vi "AvaSpec Control.vi"(6 "Path":path, 8 "error in (no error)":errorcluster, 9 "Sphere Indicator":T1, 10 "dup Message Queue":refnum<queue>, 11 "VI ref":refnum<vi>) -> (0 "error out":errorcluster)   [LabVIEW 2013]
uses:
  support/Message Queue/Message Cluster.ctl
  Acquisition/Sphere Indicator.ctl
  support/Message Queue/AvaSpec Message Queue.lvlib
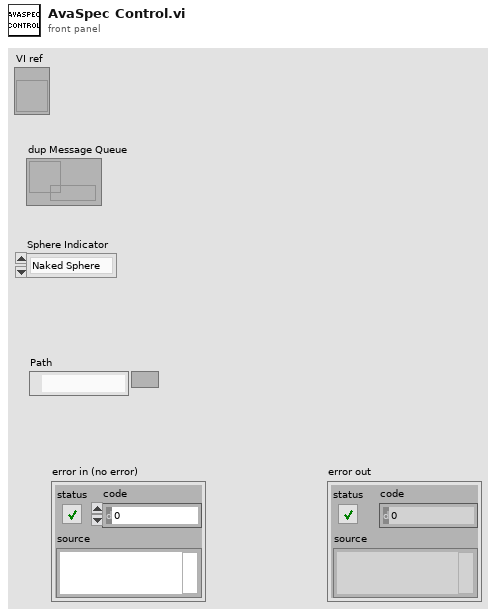
[diagram p1: front panel]
types:
  T1 = typedef "Sphere Indicator.ctl" = enum16{"Naked Sphere", "Insulated Sphere"}
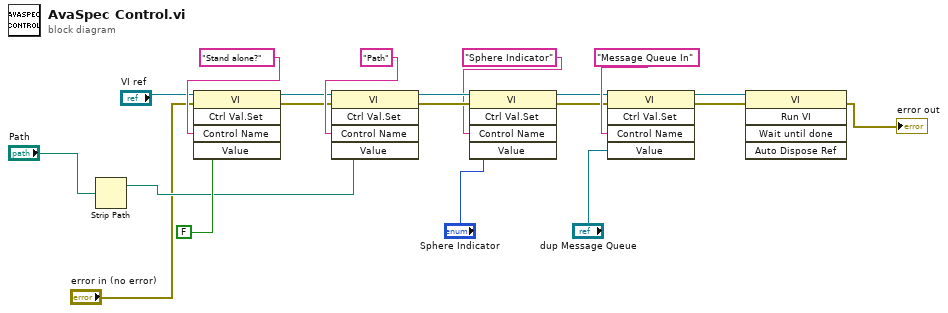
[diagram p0: block diagram]
diagram:
  n1 = Strip Path(path="Path") -> (stripped path=w4:path)  [unwired: 1 out]
  n2 = invoke class="VI" method="Ctrl Val.Set"(reference="VI ref", error in="error in (no error)", "Control Name"="Stand alone?", "Value"=FALSE) -> (reference out=w16:refnum<vi>, error out=w17:errorcluster)  [unwired: 1 in, 3 out]
  n3 = invoke class="VI" method="Ctrl Val.Set"(reference=w16, error in=w17, "Control Name"="Path", "Value"=w4) -> (reference out=w18:refnum<vi>, error out=w19:errorcluster)  [unwired: 1 in, 3 out]
  n4 = invoke class="VI" method="Ctrl Val.Set"(reference=w18, error in=w19, "Control Name"="Sphere Indicator", "Value"="Sphere Indicator") -> (reference out=w10:refnum<vi>, error out=w11:errorcluster)  [unwired: 1 in, 3 out]
  n5 = invoke class="VI" method="Ctrl Val.Set"(reference=w10, error in=w11, "Control Name"="Message Queue In", "Value"="dup Message Queue") -> (reference out=w8:refnum<vi>, error out=w7:errorcluster)  [unwired: 1 in, 3 out]
  n6 = invoke class="VI" method="Run VI"(reference=w8, error in=w7) -> (error out=→"error out":errorcluster)  [unwired: 3 in, 4 out]
